vi "XYPlot.vi"(10 "Y通道":string, 11 "X通道":string) -> ()   [LabVIEW 2018, in "DataDisplay.lvlib"]
uses:
  DataDisplay.lvlib
  XYPlot/XYPlot.lvclass
  XYPlot/XYPlotRef.ctl
  TypeDefine/DD_DataStream.ctl
  SubVI/DD_Parameter.vi
panel:
  in  "显示时长[S]":dbl=10.0 min=0.0 format="%.1f"
  in  "Y图形选择":u16(ring) items=["位移1", "力1", "次数1", "位移2", "力2", "次数2"]
  in  "X图形选择":u16(ring) items=["位移1", "力1", "次数1", "位移2", "力2", "次数2"]
  out "XY图":cluster{dbl[], dbl[]}(graph)
  # "Y轴"
  # "秒"
  # "X轴"
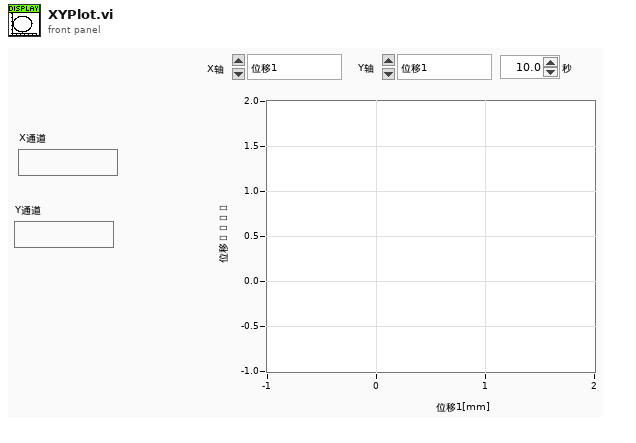
[diagram p1: front panel]
types:
  T1 = typedef "DataDisplay.lvlib/XYPlot.lvclass/XYPlotRef.ctl" = cluster{"rVI":refnum<vi>, "rPane":refnum<vi>, "rXY图":refnum<vi>, "rX通道选择":refnum<vi>, "rY通道选择":refnum<vi>, "r显示时长[S]":refnum<vi>, "DD_数据通知器":refnum<notifier>}
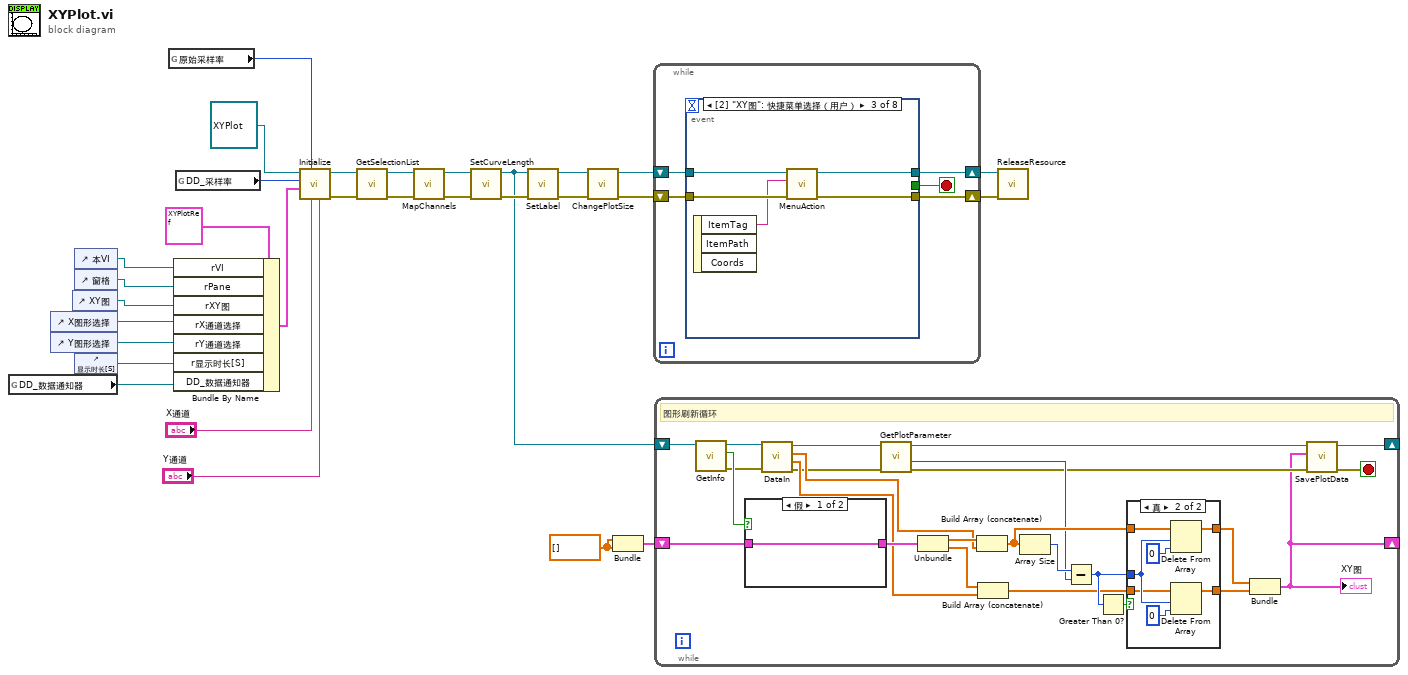
[diagram p0: block diagram]
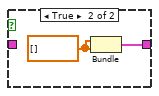
[diagram p2: hidden frame]
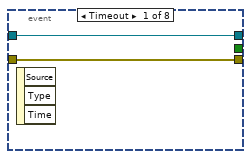
[diagram p4: hidden frame]
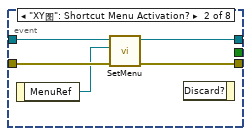
[diagram p5: hidden frame]
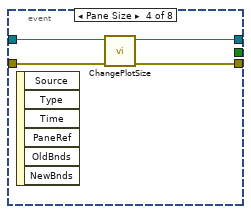
[diagram p6: hidden frame]
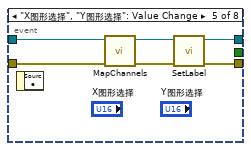
[diagram p7: hidden frame]
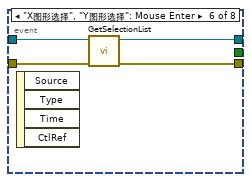
[diagram p8: hidden frame]
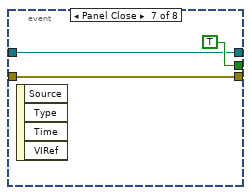
[diagram p9: hidden frame]
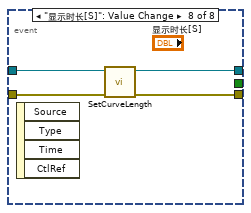
[diagram p10: hidden frame]
diagram:
  w7 = dbl[] []
  n1 = global read "DD_Parameter.vi" "DD_数据通知器"() -> (w27:refnum<notifier>)
  n2 = control-ref of="X图形选择"() -> (w24:refnum<vi>)
  n3 = control-ref of="Y图形选择"() -> (w25:refnum<vi>)
  n4 = control-ref of="XY图"() -> (w23:refnum<vi>)
  n5 = control-ref of="本VI"() -> (w21:refnum<vi>)
  n6 = control-ref of="窗格"() -> (w22:refnum<vi>)
  n7 = control-ref of="显示时长[S]"() -> (w26:refnum<vi>)
  n8 = global read "DD_Parameter.vi" "原始采样率"() -> (w3:i32)
  n9 = Bundle By Name(cluster=T1 {"rVI"=refnum, "rPane"=refnum, "rXY图"=refnum, "rX通道选择"=refnum, "rY通道选择"=refnum, "r显示时长[S]"=refnum, "DD_数据通知器"=refnum} ("引用"), "rVI"=w21, "rPane"=w22, "rXY图"=w23, "rX通道选择"=w24, "rY通道选择"=w25, "r显示时长[S]"=w26, "DD_数据通知器"=w27) -> (w20:T1)
  n10 = global read "DD_Parameter.vi" "DD_采样率"() -> (w29:i32)
  n11 = call "Initialize.vi"("Y通道"="Y通道", "X通道"="X通道", "原始采样率[Hz]"=w3, "引用"=w20, "显示采样率[Hz]"=w29, "XYPlot 输入"=refnum<class "XYPlot.lvclass"> refnum ("DataDisplay.lvlib:XYPlot.lvclass")) -> ("error out"=w18:errorcluster, "XYPlot 输出"=w8:refnum<class "XYPlot.lvclass">)  [unwired: 4 in]
  n12 = call "GetSelectionList.vi"("error in (no error)"=w18, "XYPlot 输入"=w8) -> ("error out"=w17:errorcluster, "XYPlot 输出"=w19:refnum<class "XYPlot.lvclass">)  [unwired: 8 in]
  n13 = call "MapChannels.vi"("error in (no error)"=w17, "XYPlot 输入"=w19) -> ("error out"=w16:errorcluster, "XYPlot 输出"=w5:refnum<class "XYPlot.lvclass">)  [unwired: 8 in]
  n14 = call "SetCurveLength.vi"("error in (no error)"=w16, "XYPlot 输入"=w5) -> ("error out"=w15:errorcluster, "XYPlot 输出"=w4:refnum<class "XYPlot.lvclass">)  [unwired: 8 in]
  n15 = call "SetLabel.vi"("error in (no error)"=w15, "XYPlot 输入"=w4) -> ("error out"=w10:errorcluster, "XYPlot 输出"=w12:refnum<class "XYPlot.lvclass">)  [unwired: 8 in]
  n16 = call "ChangePlotSize.vi"("error in (no error)"=w10, "XYPlot 输入"=w12) -> ("error out"=w9:errorcluster, "XYPlot 输出"=w11:refnum<class "XYPlot.lvclass">)  [unwired: 8 in]
  n17 = Bundle(w7, w7) -> (w6:cluster{dbl[], dbl[]})  [unwired: 1 in]
  n18 = while {
    shift-right: [w32] -> w14
    shift-left: w11 -> [w34]
    shift-right: [w31] -> w13
    shift-left: w9 -> [w33]
    stop <- w35 stop-if-true
    n19 = event shown="[2] \"XY图\": 快捷菜单选择（用户）" {
      selector: _ -> [_ _ _ _ _ _ _ _]
      dyn-events: _ -> [_ _ _ _ _ _ _ _]
      timeout: _ -> [_ _ _ _ _ _ _ _]
      tunnel: [_ _ _ _ _ _ TRUE _] -> w35
      tunnel: w34 -> [w37 w40 w45 w51 w57 w61 w63 w68]
      tunnel: w33 -> [w36 w42 w47 w50 w54 w60 w62 w67]
      tunnel: [w37 w39 w44 w48 w55 w59 w63 w65] -> w32
      tunnel: [w36 w41 w46 w49 w52 w58 w62 w66] -> w31
      event Timeout {
        n20 = event-data() -> ()  [unwired: 1 in, 3 out]
      }
      event "XY图": Shortcut Menu Activation? {
        n21 = event-data() -> ("MenuRef"=w38:refnum<k9>)  [unwired: 1 in]
        n22 = call "SetMenu.vi"("error in (no error)"=w42, "菜单引用"=w38, "XYPlot 输入"=w40) -> ("error out"=w41:errorcluster, "XYPlot 输出"=w39:refnum<class "XYPlot.lvclass">)  [unwired: 7 in]
        n23 = event-data() -> ()  [unwired: 2 in, 1 out]
      }
      event "XY图": Shortcut Menu Selection (User) {
        n24 = event-data() -> ("ItemTag"=w43:string)  [unwired: 1 in, 2 out]
        n25 = call "MenuAction.vi"("error in (no error)"=w47, "项标识符"=w43, "XYPlot 输入"=w45) -> ("error out"=w46:errorcluster, "XYPlot 输出"=w44:refnum<class "XYPlot.lvclass">)  [unwired: 7 in]
      }
      event Pane Size {
        n26 = event-data() -> ()  [unwired: 1 in, 6 out]
        n27 = call "ChangePlotSize.vi"("error in (no error)"=w50, "XYPlot 输入"=w51) -> ("error out"=w49:errorcluster, "XYPlot 输出"=w48:refnum<class "XYPlot.lvclass">)  [unwired: 8 in]
      }
      event "X图形选择", "Y图形选择": Value Change {
        n28 = event-data() -> ()  [unwired: 1 in, 1 out]
        n29 = call "MapChannels.vi"("error in (no error)"=w54, "XYPlot 输入"=w57) -> ("error out"=w53:errorcluster, "XYPlot 输出"=w56:refnum<class "XYPlot.lvclass">)  [unwired: 8 in]
        n30 = call "SetLabel.vi"("error in (no error)"=w53, "XYPlot 输入"=w56) -> ("error out"=w52:errorcluster, "XYPlot 输出"=w55:refnum<class "XYPlot.lvclass">)  [unwired: 8 in]
      }
      event "X图形选择", "Y图形选择": Mouse Enter {
        n31 = event-data() -> ()  [unwired: 1 in, 4 out]
        n32 = call "GetSelectionList.vi"("error in (no error)"=w60, "XYPlot 输入"=w61) -> ("error out"=w58:errorcluster, "XYPlot 输出"=w59:refnum<class "XYPlot.lvclass">)  [unwired: 8 in]
      }
      event Panel Close {
        n33 = event-data() -> ()  [unwired: 1 in, 4 out]
      }
      event "显示时长[S]": Value Change {
        n34 = event-data() -> ()  [unwired: 1 in, 4 out]
        n35 = call "SetCurveLength.vi"("error in (no error)"=w67, "XYPlot 输入"=w68) -> ("error out"=w66:errorcluster, "XYPlot 输出"=w65:refnum<class "XYPlot.lvclass">)  [unwired: 8 in]
      }
    }
  }
  n36 = while {
    shift-right: [w69] -> _
    shift-left: w6 -> [w85]
    shift-right: [w72] -> _
    shift-left: w4 -> [w88]
    stop <- w74 stop-if-true
    # "图形刷新循环"
    n37 = call "GetInfo.vi"("XYPlot 输入"=w88) -> ("error out"=w81:errorcluster, "通道变更"=w83:bool, "XYPlot 输出"=w82:refnum<class "XYPlot.lvclass">)  [unwired: 8 in]
    n38 = case shown="假" w83 {
      tunnel: w85 -> [w94 _]
      tunnel: [w94 w95] -> w84
      frame False {
      }
      frame True {
        w96 = dbl[] []
        n39 = Bundle(w96, w96) -> (w95:cluster{dbl[], dbl[]})  [unwired: 1 in]
      }
    }
    n40 = call "DataIn.vi"("error in (no error)"=w81, "XYPlot 输入"=w82) -> ("error out"=w77:errorcluster, "Data1"=w79:dbl[], "Data0"=w80:dbl[], "XYPlot 输出"=w78:refnum<class "XYPlot.lvclass">)  [unwired: 6 in]
    n41 = call "GetPlotParameter.vi"("error in (no error)"=w77, "XYPlot 输入"=w78) -> ("error out"=w75:errorcluster, "曲线点数"=w76:i32, "XYPlot 输出"=w73:refnum<class "XYPlot.lvclass">)  [unwired: 7 in]
    n42 = Unbundle(w84) -> (w87:dbl[], w86:dbl[])
    n43 = Build Array (concatenate)(w87, w80) -> (w93:dbl[])
    n44 = Build Array (concatenate)(w86, w79) -> (w89:dbl[])
    n45 = Array Size(array=w93) -> (size(s)=w92:i32)
    n46 = Subtract(x=w92, y=w76) -> (x-y=w90:i32)
    n47 = Greater Than 0?(x=w90) -> (x > 0?=w91:bool)
    n48 = case shown="真" w91 {
      tunnel: w93 -> [w98 w105]
      tunnel: w90 -> [_ w101]
      tunnel: [w98 w103] -> w71
      tunnel: w89 -> [w97 w100]
      tunnel: [w97 w99] -> w70
      frame False {
      }
      frame True {
        n49 = Delete From Array(array=w105, length=w101, index=0 ("索引")) -> (array with subset deleted=w103:dbl[])  [unwired: 1 out]
        n50 = Delete From Array(array=w100, length=w101, index=0 ("索引")) -> (array with subset deleted=w99:dbl[])  [unwired: 1 out]
      }
    }
    n51 = Bundle(w71, w70) -> (w69:cluster{dbl[], dbl[]})  [unwired: 1 in]
    "XY图" <- w69
    n52 = call "SavePlotData.vi"("error in (no error)"=w75, "数据输入"=w69, "XYPlot 输入"=w73) -> ("error out"=w74:errorcluster, "XYPlot 输出"=w72:refnum<class "XYPlot.lvclass">)  [unwired: 7 in]
  }
  n53 = call "ReleaseResource.vi"("error in (no error)"=w13, "XYPlot 输入"=w14) -> ()  [unwired: 8 in, 2 out]
